vi "OP500_Scan Array.vi"(11 "Array":dbl[](array[numeric])) -> (3 "Indice du premier valeur du courant DCIR":i32)   [LabVIEW 2020]
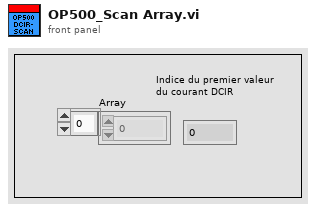
[diagram p1: front panel]
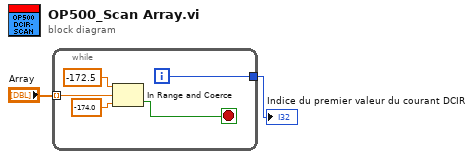
[diagram p0: block diagram]
diagram:
  n1 = while {
    tunnel: "Array" -> [w5] mode=indexing
    tunnel: [w4] -> w2
    i -> [w4]
    stop <- w3 stop-if-true
    n2 = In Range and Coerce(upper limit=-172.5, x=w5, lower limit=-174.0) -> (In Range?=w3:bool)  [unwired: 1 out]
  }
  "Indice du premier valeur du courant DCIR" <- w2
